vi "Control_temp.vi"() -> ()   [LabVIEW 2019]
uses:
  Control_temp.ctl
panel:
  in  "Rata de T":T1=1.0 scale=0.0..10.0
  out "Sensor de temperatura en °C":dbl(slide) scale=0.0..100.0
  in  "Selector":bool
  # "Incrementar\n\nDecrementar"
  # "Rata T(5°C/seg)"
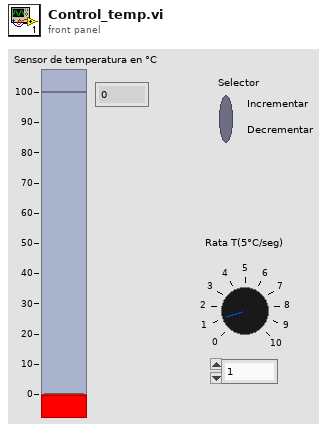
[diagram p1: front panel]
types:
  T1 = typedef "Control_temp.ctl" = dbl
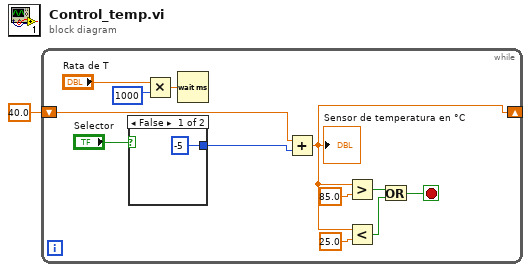
[diagram p0: block diagram]
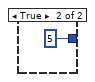
[diagram p2: hidden frame]
diagram:
  n1 = while {
    shift-right: [w7] -> _
    shift-left: T1 40.0 ("Rata de T") -> [w12]
    stop <- w9 stop-if-true
    n2 = case shown="False" "Selector" {
      tunnel: [-5 5] -> w5
      frame False {
      }
      frame True {
      }
    }
    n3 = Multiply(x="Rata de T", y=1000) -> (x*y=w4:T1)
    n4 = Wait (ms)(milliseconds to wait=w4) -> ()  [unwired: 1 out]
    n5 = Add(x=w12, y=w5) -> (x+y=w7:T1)
    "Sensor de temperatura en °C" <- w7
    n6 = Greater?(x=w7, y=85.0) -> (0:w11:bool)
    n7 = Less?(x=w7, y=T1 25.0) -> (x < y?=w10:bool)
    n8 = Or(x=w11, y=w10) -> (x .or. y?=w9:bool)
  }
